vi "Create.vi"(8 "error in (no error)":errorcluster, 11 "Record":variant[](array[variant])) -> (0 "error out":errorcluster, 3 "Category out":refnum<class "Category.lvclass">)   [LabVIEW 2018, in "Category.lvclass"]
uses:
  Category.lvclass
  Category.lvclass/Category.ctl
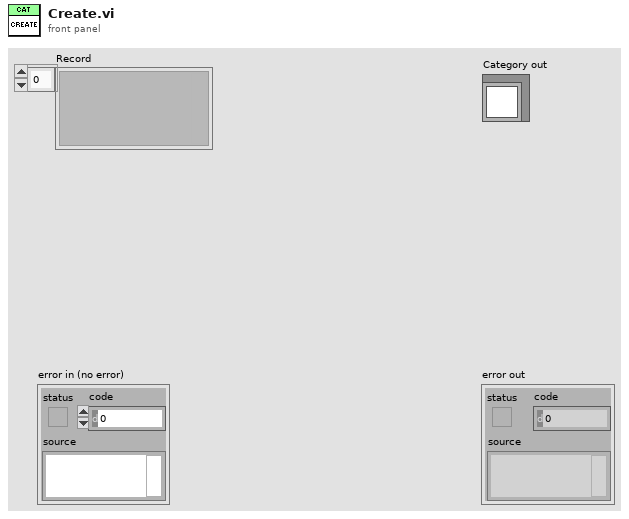
[diagram p1: front panel]
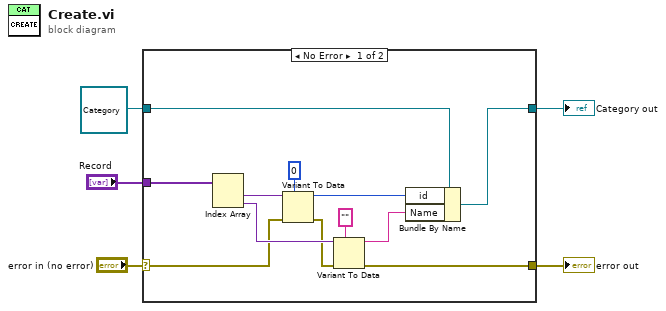
[diagram p0: block diagram]
diagram:
  n1 = case shown="No Error" "error in (no error)" {
    selector: "error in (no error)" -> [w8 w19]
    tunnel: [w6 w19] -> w4
    tunnel: [w13 w18] -> w2
    tunnel: refnum<class "Category.lvclass"> refnum ("Category in") -> [w14 w18]
    tunnel: "Record" -> [w17 _]
    frame No Error {
      n2 = Index Array(array=w17) -> (element #1=w16:variant, element #2=w15:variant)  [unwired: 2 in]
      n3 = Variant To Data(error in=w8, type=0, Variant=w16) -> (data=w11:i32, error out=w7:errorcluster)
      n4 = Variant To Data(error in=w7, type="", Variant=w15) -> (data=w9:string, error out=w6:errorcluster)
      n5 = Bundle By Name(cluster=w14, "id"=w11, "Name"=w9) -> (w13:refnum<class "Category.lvclass">)
    }
    frame Error {
    }
  }
  "error out" <- w4
  "Category out" <- w2
